vi "HTTP GET.vi"(6 "request specific headers":T1[](array[typedef]), 7 "timeout (0 = Use Default)":i32, 8 "error in (no error)":errorcluster, 10 "Path":string, 11 "REST Client_NET in":refnum<class "REST Client_NET.lvclass">) -> (0 "error out":errorcluster, 1 "Response body":string, 2 "Response Headers":refnum<class "Response Headers.lvclass">, 3 "REST Client_NET out":refnum<class "REST Client_NET.lvclass">, 4 "Status String":string, 5 "Status Code":u16)   [LabVIEW 2018, in "REST Client_NET.lvlib" / "REST Client_NET.lvclass"]
doc: "Perform a HTTP GET request.\n\nThe VI provides multiple arguments for defining how to perform the HTTP request.\n\n<b>Path</b> specifies the path beneath the Base URL to be used for the HTTP request.\nrequest specific headers specifies an array of headers to be used with this particular HTTP request. \n\n<b>request specific headers</b> The Default Headers specified upon creation of the JKI REST Client together with the request specific headers will all be used for the HTTP request.\n<b> </b> <b> </b>\nHttpClient_NET\nJustin Young - Viviota\nCopyright (c) 2021\nLicense: BSD"
uses:
  REST Client_NET.lvclass
  <vilib>/addons/_JKI.lib/REST Client/classes/Response Headers/Response Headers.lvclass
  <vilib>/addons/_JKI.lib/REST Client/classes/REST Client/HTTP Header.ctl
  <vilib>/addons/_JKI.lib/REST Client/classes/REST Client/HTTP Methods.ctl
  <vilib>/addons/_JKI.lib/REST Client/classes/REST Client/REST Client.lvclass
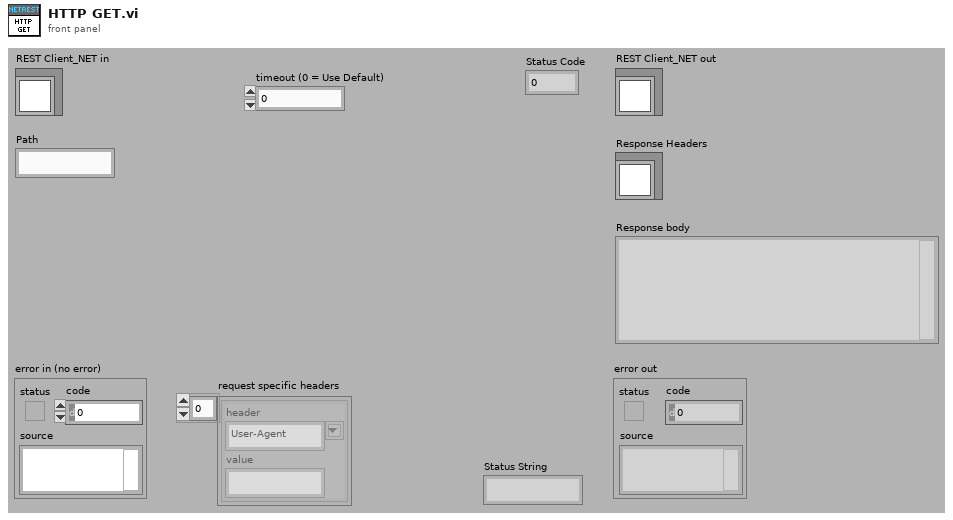
[diagram p1: front panel]
types:
  T1 = typedef "REST Client.lvlib/REST Client.lvclass/HTTP Header.ctl" = cluster{"header":string, "value":string}
  T2 = typedef "REST Client.lvlib/REST Client.lvclass/HTTP Methods.ctl" = enum16{"GET", "HEAD", "POST", "PUT", "DELETE"}
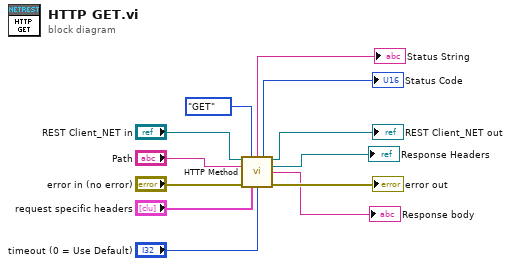
[diagram p0: block diagram]
diagram:
  n1 = call "HTTP Method.vi"("REST Client_NET in"="REST Client_NET in", "Method"=HTTP_Methods."GET", "Path"="Path", "error in (no error)"="error in (no error)", "request specific headers"="request specific headers", "timeout (0 = Use Default)"="timeout (0 = Use Default)") -> ("ReasonPhrase"=→"Status String":string, "StatusCode"=→"Status Code":i32, "REST Client_NET out"=→"REST Client_NET out":refnum<class "REST Client_NET.lvclass">, "Response Headers out"=→"Response Headers":refnum<class "Response Headers.lvclass">, "Response"=→"Response body":string, "error out"=→"error out":errorcluster)  [unwired: 4 in]
